vi "AB_RW_Project_DLL_Info.vi"(7 "action":T1, 8 "error in (no error)":errorcluster, 10 "Dll_info in":T2, 11 "Object In":T3) -> (0 "error out":errorcluster, 2 "Dll info out":T2, 3 "Object Out":T3)   [LabVIEW 2020]
uses:
  <resource>/Framework/Providers/API/ItemRef.ctl
  <vilib>/AppBuilder/RW_Project/AB_RW_Project_DLL_Data.ctl
  <vilib>/AppBuilder/RW_Project/AB_RW_Project_PropBag_Action.ctl
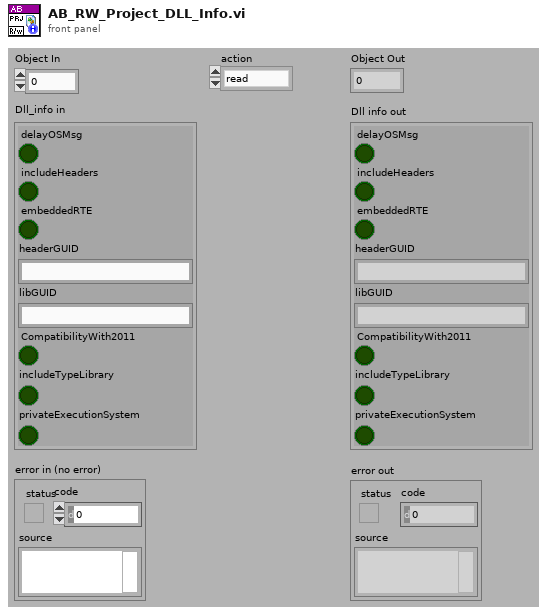
[diagram p1: front panel]
types:
  T1 = typedef "AB_RW_Project_PropBag_Action.ctl" = enum16{"read", "write", "clear", "readPrevious", "writePrevious", "clearPrevious"}
  T2 = typedef "AB_RW_Project_DLL_Data.ctl" = cluster{"delayOSMsg":bool, "includeHeaders":bool, "embeddedRTE":bool, "headerGUID":string, "libGUID":string, "CompatibilityWith2011":bool, "includeTypeLibrary":bool, "privateExecutionSystem":bool}
  T3 = typedef "ItemRef.ctl" = u64
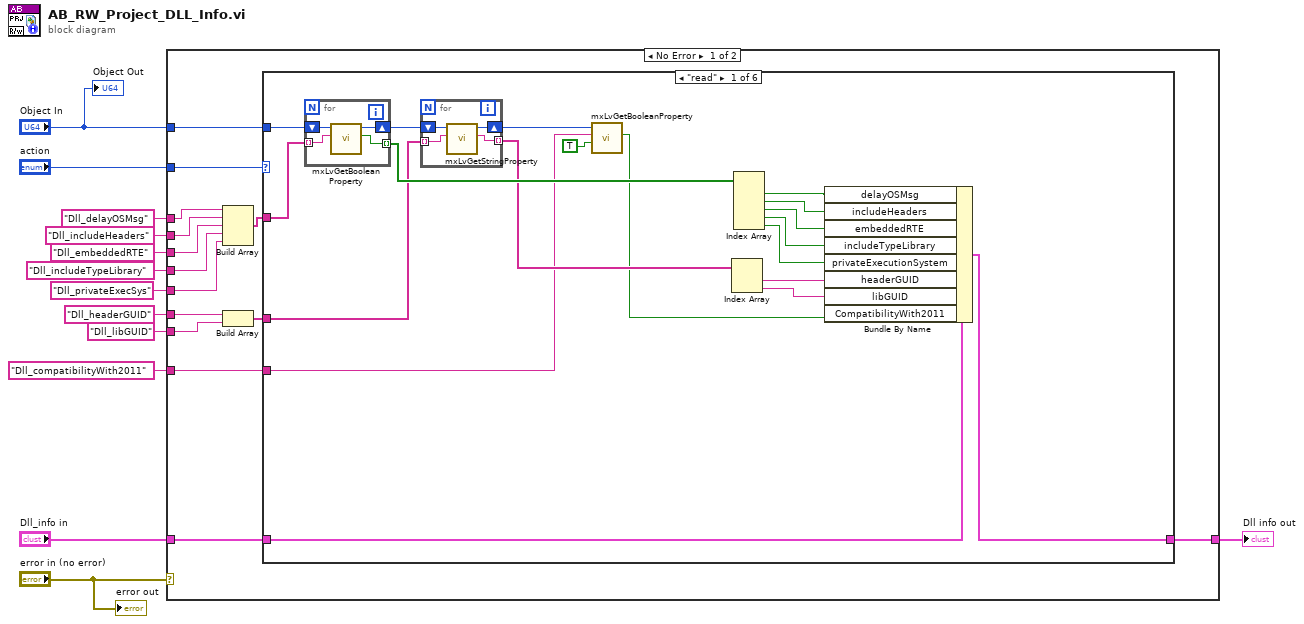
[diagram p0: block diagram]
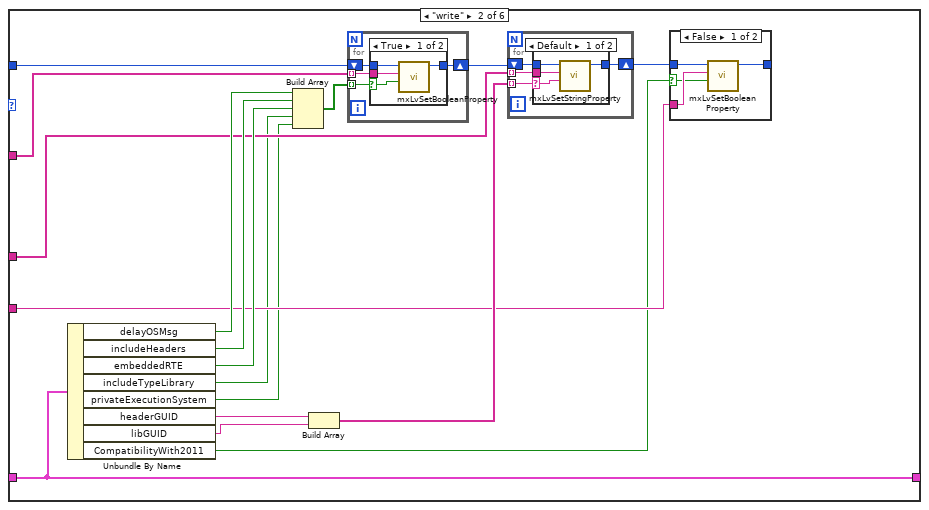
[diagram p2: hidden frame]
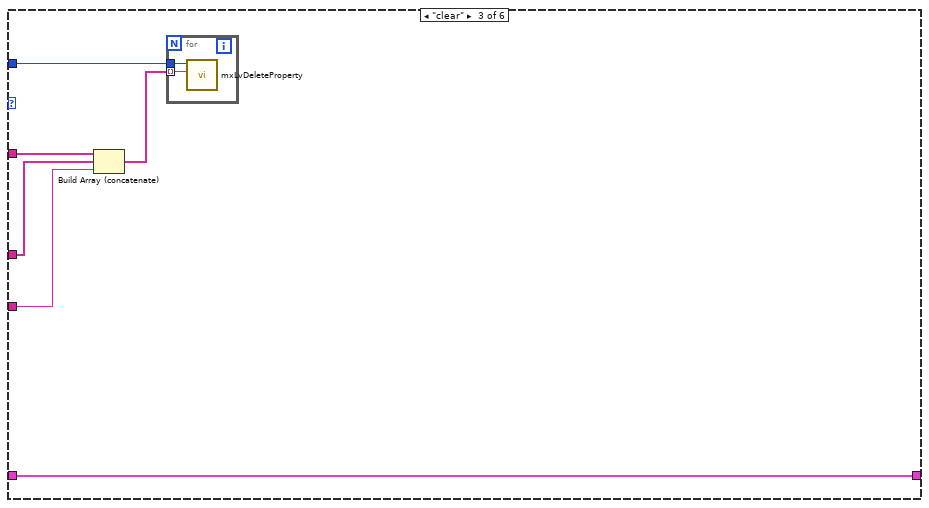
[diagram p6: hidden frame]
diagram:
  n1 = case shown="No Error" "error in (no error)" {
    tunnel: "Object In" -> [w26 _]
    tunnel: [w27 _] -> w11
    tunnel: "Dll_info in" -> [w25 _]
    tunnel: "action" -> [w24 _]
    tunnel: "Dll_delayOSMsg" -> [w23 _]
    tunnel: "Dll_includeHeaders" ("Tag") -> [w22 _]
    tunnel: "Dll_embeddedRTE" ("Tag") -> [w21 _]
    tunnel: "Dll_headerGUID" -> [w20 _]
    tunnel: "Dll_libGUID" -> [w19 _]
    tunnel: "Dll_compatibilityWith2011" -> [w16 _]
    tunnel: "Dll_includeTypeLibrary" -> [w15 _]
    tunnel: "Dll_privateExecSys" -> [w14 _]
    frame No Error {
      n2 = Build Array(w23, w22, w21, w15, w14) -> (w18:string[])
      n3 = Build Array(w20, w19) -> (w17:string[])
      n4 = case shown="\"read\"" w24 {
        tunnel: [w35 w62 w100 w103 w104 w105] -> w27
        tunnel: w26 -> [w33 w63 w99 _ _ _]
        tunnel: w25 -> [w36 w62 w100 w103 w104 w105]
        tunnel: w18 -> [w38 w61 w97 _ _ _]
        tunnel: w17 -> [w37 w60 w96 _ _ _]
        tunnel: w16 -> [w34 w59 w95 _ _ _]
        frame "read" {
          n5 = for {
            shift-right: [w53] -> w46
            shift-left: w33 -> [w54]
            tunnel: [w52] -> w45 mode=indexing
            tunnel: w38 -> [w51] mode=indexing
            n6 = call <resource>:"mxLvGetBooleanProperty.vi"("Tag"=w51, "Item"=w54) -> ("Value"=w52:bool, "Item"=w53:T3)  [unwired: 7 in, 1 out]
          }
          n7 = for {
            shift-right: [w49] -> w30
            shift-left: w46 -> [w50]
            tunnel: [w48] -> w41 mode=indexing
            tunnel: w37 -> [w47] mode=indexing
            n8 = call <resource>:"mxLvGetStringProperty.vi"("Tag"=w47, "Item"=w50) -> ("Value"=w48:string, "Item"=w49:T3)  [unwired: 7 in, 1 out]
          }
          n9 = call <resource>:"mxLvGetBooleanProperty.vi"("Default Value (F)"=TRUE, "Tag"=w34, "Item"=w30) -> ("Value"=w31:bool)  [unwired: 6 in, 2 out]
          n10 = Index Array(array=w41) -> (element #1=w40:string, element #2=w39:string)  [unwired: 2 in]
          n11 = Index Array(array=w45) -> (element #1=w44:bool, element #2=w43:bool, element #3=w42:bool, element #4=w29:bool, element #5=w28:bool)  [unwired: 5 in]
          n12 = Bundle By Name(cluster=w36, "delayOSMsg"=w44, "includeHeaders"=w43, "embeddedRTE"=w42, "includeTypeLibrary"=w29, "privateExecutionSystem"=w28, "headerGUID"=w40, "libGUID"=w39, "CompatibilityWith2011"=w31) -> (w35:T2)
        }
        frame "write" {
          n13 = Unbundle By Name(w62) -> ("delayOSMsg"=w71:bool, "includeHeaders"=w70:bool, "embeddedRTE"=w69:bool, "includeTypeLibrary"=w56:bool, "privateExecutionSystem"=w55:bool, "headerGUID"=w67:string, "libGUID"=w66:string, "CompatibilityWith2011"=w58:bool)
          n14 = Build Array(w71, w70, w69, w56, w55) -> (w68:bool[])
          n15 = Build Array(w67, w66) -> (w64:string[])
          n16 = for {
            tunnel: w68 -> [w88] mode=indexing
            shift-right: [w87] -> w65
            shift-left: w63 -> [w89]
            tunnel: w61 -> [w86] mode=indexing
            n17 = case shown="True" w88 {
              selector: w88 -> [w92 _]
              tunnel: w89 -> [w93 w94]
              tunnel: w86 -> [w90 _]
              tunnel: [w91 w94] -> w87
              frame True {
                n18 = call <resource>:"mxLvSetBooleanProperty.vi"("Value (F)"=w92, "Tag"=w90, "Item"=w93) -> ("Item"=w91:T3)  [unwired: 7 in, 1 out]
              }
              frame False {
              }
            }
          }
          n19 = for {
            tunnel: w64 -> [w79] mode=indexing
            shift-right: [w78] -> w57
            shift-left: w65 -> [w80]
            tunnel: w60 -> [w77] mode=indexing
            n20 = case shown="Default" w79 {
              selector: w79 -> [w82 _]
              tunnel: w80 -> [w84 w85]
              tunnel: w77 -> [w81 _]
              tunnel: [w83 w85] -> w78
              frame Default {
                n21 = call <resource>:"mxLvSetStringProperty.vi"("Value (\"\")"=w82, "Tag"=w81, "Item"=w84) -> ("Item"=w83:T3)  [unwired: 7 in, 1 out]
              }
              frame "" {
              }
            }
          }
          n22 = case shown="False" w58 {
            selector: w58 -> [w73 _]
            tunnel: w59 -> [w75 _]
            tunnel: w57 -> [w74 w76]
            tunnel: [w72 w76] -> _
            frame False {
              n23 = call <resource>:"mxLvSetBooleanProperty.vi"("Value (F)"=w73, "Tag"=w75, "Item"=w74) -> ("Item"=w72:T3)  [unwired: 7 in, 1 out]
            }
            frame True {
            }
          }
        }
        frame "clear" {
          n24 = Build Array (concatenate)(w97, w96, w95) -> (w98:string[])
          n25 = for {
            tunnel: w99 -> [w102]
            tunnel: w98 -> [w101] mode=indexing
            n26 = call <resource>:"mxLvDeleteProperty.vi"("Tag"=w101, "Item"=w102) -> ()  [unwired: 8 in, 2 out]
          }
        }
        frame "readPrevious" {
        }
        frame "writePrevious" {
        }
        frame "clearPrevious" {
        }
      }
    }
    frame Error {
    }
  }
  "Dll info out" <- w11
  "Object Out" <- "Object In"
  "error out" <- "error in (no error)"
